vi "IMAGEExample_S.vi"(1 "Image":T1) -> (0 "String":string)   [LabVIEW 2019]
doc: "Determines where the image will be saved and the image name used (e.g IMG12313123_2542.PNG)"
uses:
  <vilib>/vision/Image Controls.llb/IMAQ Image.ctl
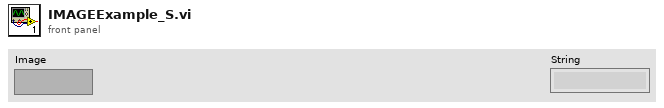
[diagram p1: front panel]
types:
  T1 = typedef "IMAQ Image.ctl" = refnum<image>
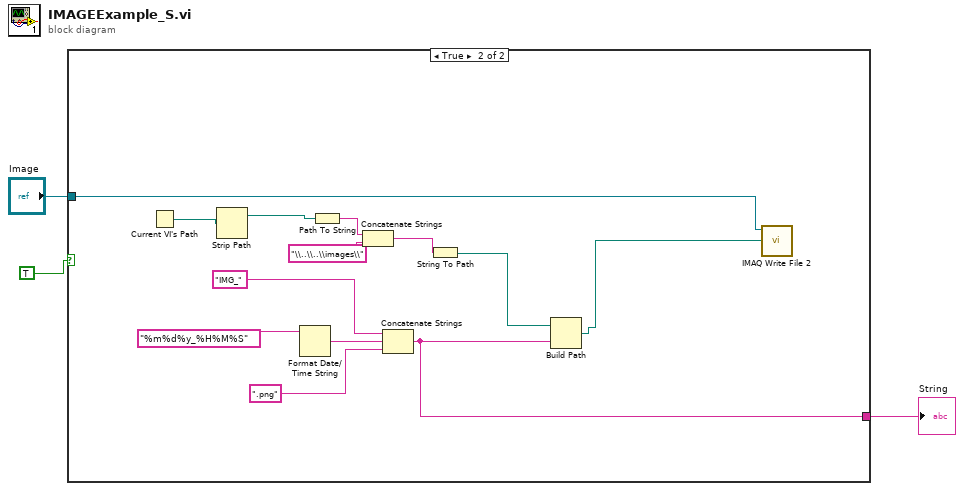
[diagram p0: block diagram]
diagram:
  n1 = case shown="True" TRUE {
    tunnel: "Image" -> [_ w5]
    tunnel: [_ w4] -> w1
    frame False {
    }
    frame True {
      n2 = Current VI's Path() -> (path=w12:path)
      n3 = Strip Path(path=w12) -> (stripped path=w11:path)  [unwired: 1 out]
      n4 = Format Date/Time String(time format string (%c)="%m%d%y_%H%M%S") -> (date/time string=w14:string)  [unwired: 2 in]
      n5 = Path To String(path=w11) -> (string=w8:string)
      n6 = Concatenate Strings(w8, "\\..\\..\\images\\") -> (w7:string)
      n7 = Concatenate Strings("IMG_", w14, ".png") -> (w4:string)
      n8 = String To Path(string=w7) -> (path=w10:path)
      n9 = Build Path(base path=w10, name or relative path=w4) -> (appended path=w6:path)
      n10 = call-poly "IMAQ Write File 2"("File Path"=w6, "Image"=w5) -> ()  [unwired: 8 in, 2 out]
    }
  }
  "String" <- w1
